vi "Error.vi"(8 "error in":errorcluster, 11 "Ignore Errors (Runtime)":i32[](array[numeric])) -> (0 "error out":errorcluster)   [LabVIEW 2014]
uses:
  Message Queue/Message Queue.lvlib
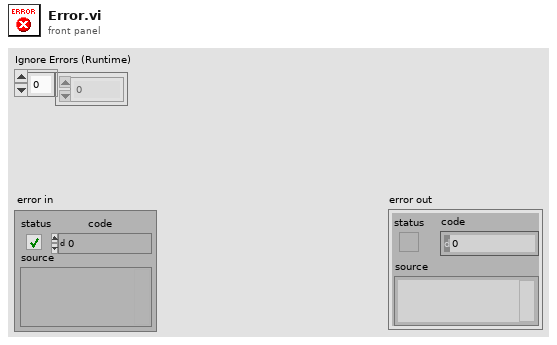
[diagram p1: front panel]
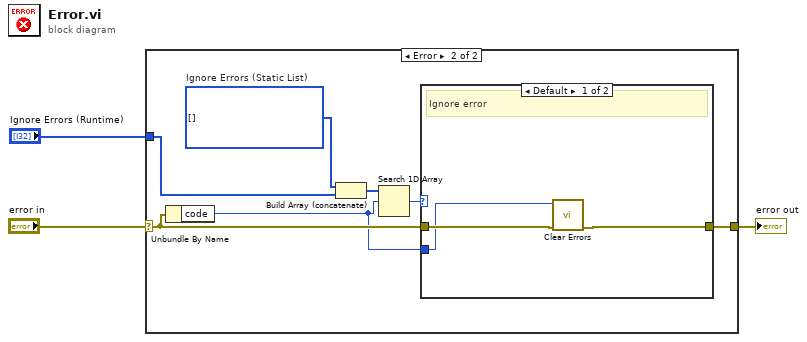
[diagram p0: block diagram]
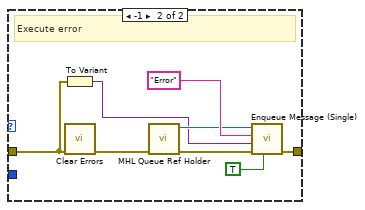
[diagram p3: hidden frame]
diagram:
  n1 = case shown="Error" "error in" {
    selector: "error in" -> [w4 w7]
    tunnel: [w4 w11] -> w3
    tunnel: "Ignore Errors (Runtime)" -> [_ w8]
    frame No Error {
    }
    frame Error {
      w9 = i32[] []  # Ignore Errors (Static List)
      n2 = Unbundle By Name(w7) -> ("code"=w5:i32)
      n3 = Build Array (concatenate)(w9, w8) -> (w10:i32[])
      n4 = Search 1D Array(1D array=w10, element=w5) -> (index of element=w6:i32)  [unwired: 1 in]
      n5 = case shown="Default" w6 {
        tunnel: w7 -> [w14 w17]
        tunnel: [w13 w15] -> w11
        tunnel: w5 -> [w12 _]
        frame Default {
          # "Ignore error"
          n6 = call <vilib>:"Clear Errors.vi"("error in (no error)"=w14, "specific error code to clear (0: all)"=w12) -> ("error out"=w13:errorcluster)  [unwired: 4 in, 1 out]
        }
        frame -1 {
          # "Execute error"
          n7 = To Variant(anything=w17) -> (Variant=w19:variant)
          n8 = call <vilib>:"Clear Errors.vi"("error in (no error)"=w17) -> ("error out"=w16:errorcluster)  [unwired: 5 in, 1 out]
          n9 = call "MHL Queue Ref Holder.vi"("error in"=w16) -> ("error out"=w20:errorcluster, "Input Message Queue"=w21:refnum<queue>)  [unwired: 9 in]
          n10 = call "Enqueue Message (Single).vi"("Priority Message? (F)"=TRUE, "error in (no error)"=w20, "Message Data"=w19, "Message"="Error", "Message Queue"=w21) -> ("error out"=w15:errorcluster)  [unwired: 5 in, 1 out]
        }
      }
    }
  }
  "error out" <- w3
